vi "Read Shift Schedule from File.vi"(8 "error in (no error)":errorcluster, 10 "XML File Path":path, 11 "Shift Schedule in":refnum<class "Shift Schedule.lvclass">) -> (0 "error out":errorcluster, 3 "Shift Schedule out":refnum<class "Shift Schedule.lvclass">)   [LabVIEW 2013]
uses:
  Shift Schedule.lvclass
  <vilib>/Utility/xml.llb/Read From XML File(string).vi
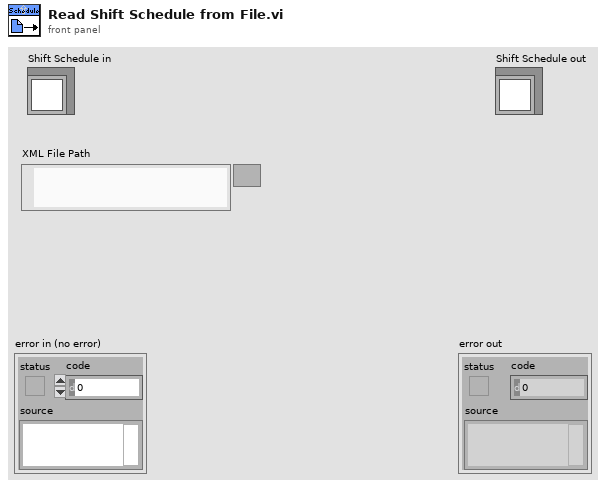
[diagram p1: front panel]
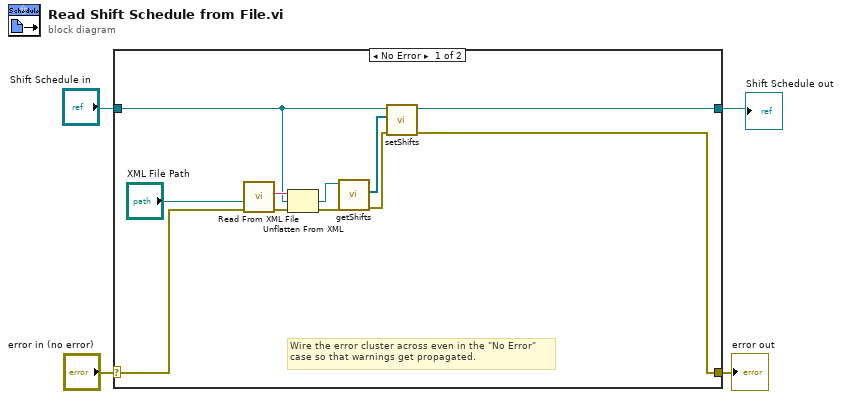
[diagram p0: block diagram]
diagram:
  n1 = case shown="No Error" "error in (no error)" {
    selector: "error in (no error)" -> [w14 w17]
    tunnel: [w7 w17] -> w3
    tunnel: [w8 w16] -> w2
    tunnel: "Shift Schedule in" -> [w6 w16]
    frame No Error {
      # "Wire the error cluster across even in the \"No Error\"\ncase so that warnings get propagated."
      n2 = call-poly <vilib>:"Read From XML File.vi"("error in (no error)"=w14, "XML File Path"="XML File Path") -> ("error out"=w13:errorcluster, "XML Elements"=w12:string)  [unwired: 7 in, 1 out]
      n3 = Unflatten From XML(xml string=w12, type=w6, error in (no error)=w13) -> (value=w10:refnum<class "Shift Schedule.lvclass">, error out=w11:errorcluster)
      n4 = call-dynamic "getShifts.vi"("error in (no error)"=w11, "Shift Schedule in"=w10) -> ("error out"=w9:errorcluster, "shifts"=w5:refnum<class "Shift.lvclass">[])  [unwired: 7 in, 1 out]
      n5 = call-dynamic "setShifts.vi"("error in (no error)"=w9, "shifts"=w5, "Shift Schedule in"=w6) -> ("error out"=w7:errorcluster, "Shift Schedule out"=w8:refnum<class "Shift Schedule.lvclass">)  [unwired: 7 in]
    }
    frame Error {
    }
  }
  "error out" <- w3
  "Shift Schedule out" <- w2
